vi "WinCI Reset Command Options.vi"(8 "error in (no error)":errorcluster) -> (0 "error out":errorcluster)   [LabVIEW 2020, in "NI_SCC_WinCI.lvlib"]
uses:
  <vilib>/SourceControl/Providers/WinCI/NI_SCC_WinCI.lvlib
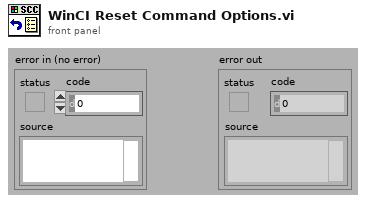
[diagram p1: front panel]
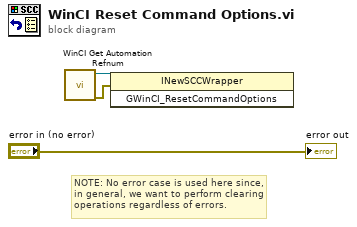
[diagram p0: block diagram]
diagram:
  # "NOTE: No error case is used here since, in general, we want to perform clearing operations regardless of errors."
  n1 = call <vilib>:"WinCI Get Automation Refnum.vi"() -> ("error out"=w2:errorcluster, "automation refnum"=w1:refnum<k7>)  [unwired: 10 out]
  n2 = invoke class="INewSCCWrapper" method="GWinCI_ResetCommandOptions"(reference=w1, error in=w2) -> ()  [unwired: 1 in, 3 out]
  "error out" <- "error in (no error)"
